vi "Update Values Buffer.vi"(8 "error in (no error)":errorcluster, 9 "buffer data":T1={"decimation"=0, "avg bandwidth"=0.0, "channels"=[], "byte order"=enum."little-endian", "buffer descriptor"={"buffer type"=enum."Engine", "plugin id"=0, "group id"=0, "transfer id"=0, "offset"=0, "length"=0}, "values channels"={"index"=0, "count"=0, "engine offset"=0}, "select start offset"=18446744073709551615, "select end offset"=0, "channel index"=-1} {"channels"."configuration"."string offset" format="%d bytes"; "avg bandwidth" format="%.0g bytes"}, 10 "buffer in":u8[](array[numeric]), 11 "values buffer in":u8[](array[numeric])) -> (0 "error out":errorcluster, 2 "buffer out":u8[](array[numeric]), 3 "values buffer out":u8[](array[numeric]))   [LabVIEW 2017, in "Data Viewer.lvlib"]
uses:
  Core/VIs/Data Viewer/Source/Data Viewer.lvlib
  Buffer Reader/Buffer Data.ctl
  VeriStand/Data Sharing Custom Device/Source/DSF Core.lvlibp/Classes/Configuration/Core/Transfer/Channel Configuration.ctl
  VeriStand/Data Sharing Custom Device/Source/DSF Core.lvlibp/Typedefs/Core Channel Configuration.ctl
  VeriStand/Data Sharing Custom Device/Source/DSF Core.lvlibp/Typedefs/DSF Data Type.ctl
  VeriStand/Data Sharing Custom Device/Source/DSF Core.lvlibp/Typedefs/DSF Settings Info.ctl
  VeriStand/Data Sharing Custom Device/Source/DSF Core.lvlibp/Typedefs/DSF Byte Order.ctl
  VeriStand/Data Sharing Custom Device/Source/DSF Core.lvlibp/Classes/Thread/Data Server/DSF Buffer Subset Descriptor.ctl
  VeriStand/Data Sharing Custom Device/Source/DSF Core.lvlibp/Typedefs/DSF Buffer Type.ctl
  Values Channels.ctl
  VeriStand/Data Sharing Custom Device/Source/DSF Core.lvlibp/Classes/Framework/Framework.lvclass
  VeriStand/Data Sharing Custom Device/Source/DSF Core.lvlibp
  VeriStand/Data Sharing Custom Device/Source/DSF Core.lvlibp/Classes/Configuration/Core/Channel/Channel Configuration.lvclass
  VeriStand/Data Sharing Custom Device/Source/DSF Core.lvlibp/Classes/Configuration/Core/Transfer/Transfer Configuration.lvclass
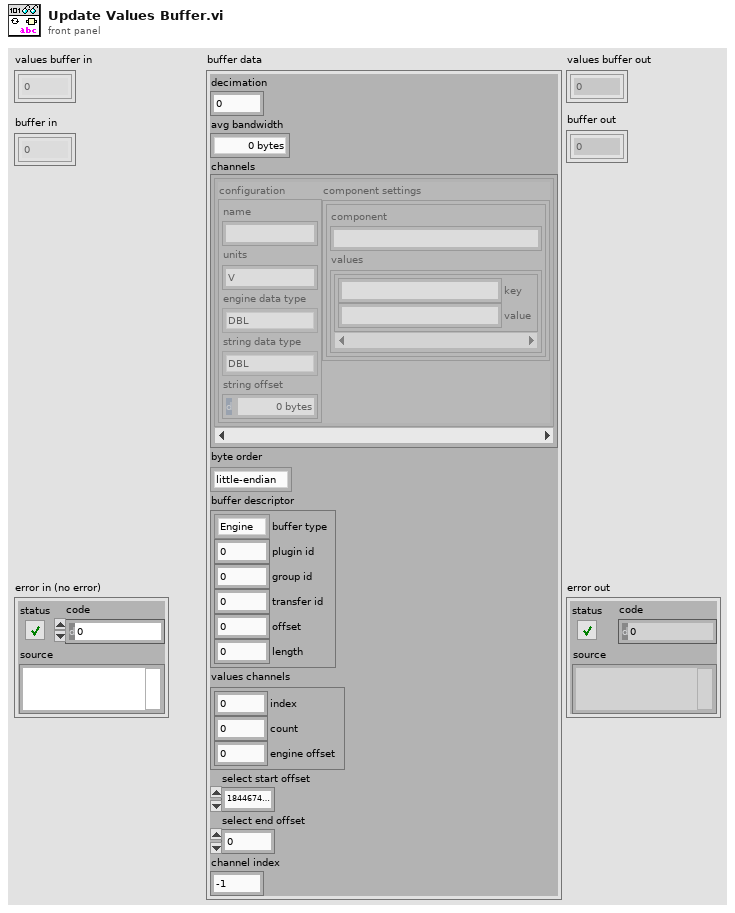
[diagram p1: front panel]
types:
  T1 = typedef "Data Viewer.lvlib/Buffer Data.ctl" = cluster{"decimation":u64, "avg bandwidth":dbl, "channels":T2[], "byte order":T6, "buffer descriptor":T7, "values channels":T9, "select start offset":u64, "select end offset":u64, "channel index":i32}
  T2 = typedef "DSF Core.lvlibp/Transfer Configuration.lvclass/Channel Configuration.ctl" = cluster{"configuration":T3, "component settings":T5[]}
  T3 = typedef "DSF Core.lvlibp/Channel Configuration.lvclass/Core Channel Configuration.ctl" = cluster{"name":string, "units":string, "engine data type":T4, "string data type":T4, "string offset":u64}
  T4 = typedef "DSF Core.lvlibp/DSF Data Type.ctl" = enum8{"Bool", "SGL", "DBL", "I8", "I16", "I32", "I64", "U8", "U16", "U32", "U64"}
  T5 = typedef "DSF Core.lvlibp/DSF Settings Info.ctl" = cluster{"component":string, "values":cluster{"key":string, "value":string}[]}
  T6 = typedef "DSF Core.lvlibp/DSF Byte Order.ctl" = enum8{"big-endian", "little-endian"}
  T7 = typedef "DSF Core.lvlibp/DSF Buffer Subset Descriptor.ctl" = cluster{"buffer type":T8, "plugin id":i32, "group id":i32, "transfer id":i32, "offset":u64, "length":i64}
  T8 = typedef "DSF Core.lvlibp/DSF Buffer Type.ctl" = enum16{"Engine", "String"}
  T9 = typedef "Data Viewer.lvlib/Values Channels.ctl" = cluster{"index":i32, "count":i32, "engine offset":u64}
  T10 = enum16{"big-endian, network order", "native, host order", "little-endian"}
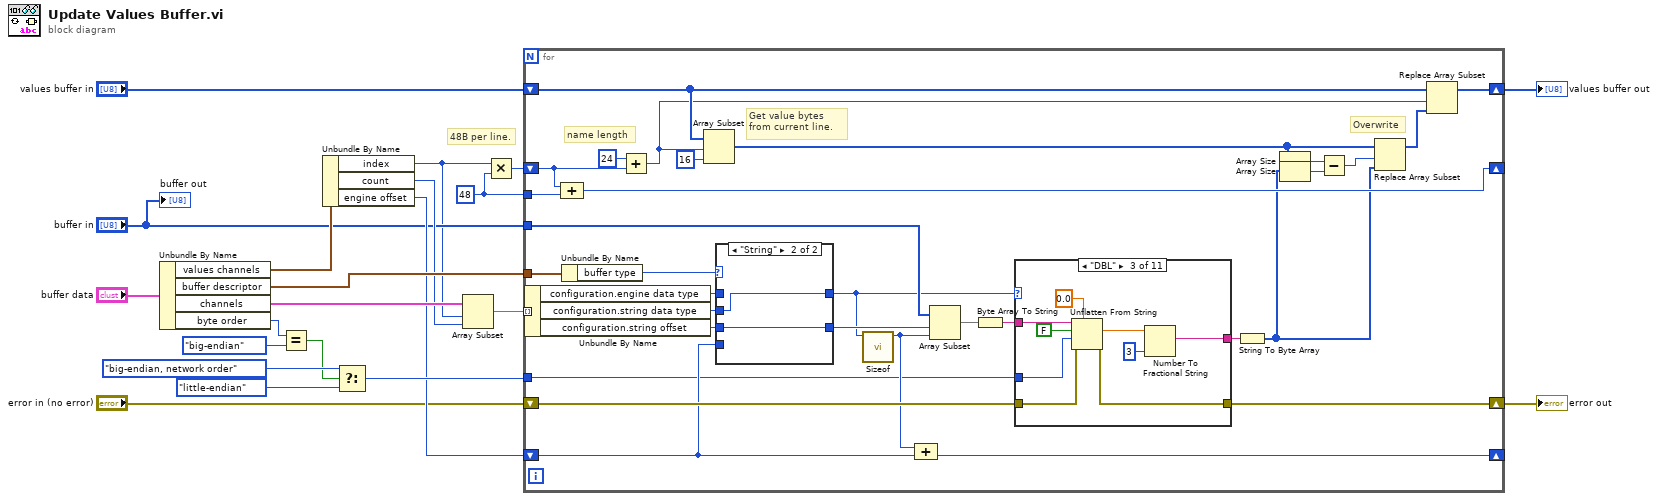
[diagram p0: block diagram]
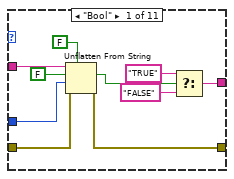
[diagram p3: hidden frame]
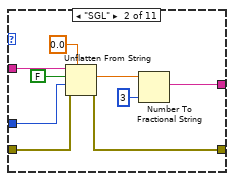
[diagram p4: hidden frame]
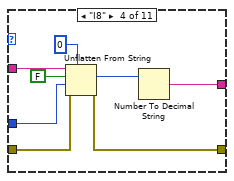
[diagram p5: hidden frame]
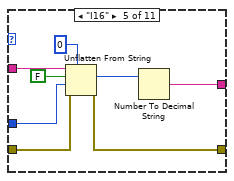
[diagram p6: hidden frame]
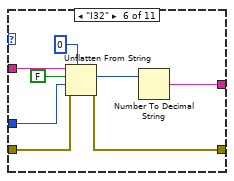
[diagram p7: hidden frame]
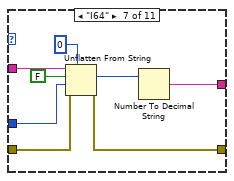
[diagram p8: hidden frame]
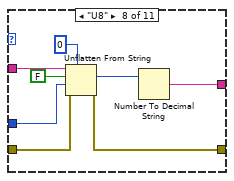
[diagram p9: hidden frame]
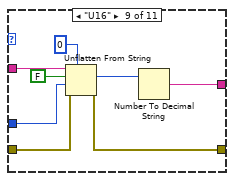
[diagram p10: hidden frame]
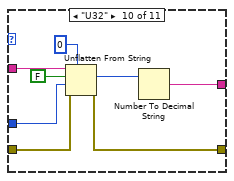
[diagram p11: hidden frame]
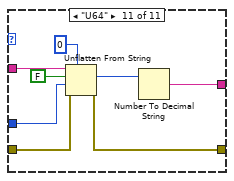
[diagram p12: hidden frame]
diagram:
  w1 = 48 ("x")
  # "48B per line."
  n1 = Unbundle By Name("buffer data") -> ("values channels"=w19:T9, "buffer descriptor"=w18:T7, "channels"=w17:T2[], "byte order"=w9:T6)
  n2 = Equal?(x=w9, y=DSF_Byte_Order."big-endian") -> (x = y?=w5:bool)
  n3 = Unbundle By Name(w19) -> ("index"=w2:i32, "count"=w10:i32, "engine offset"=w7:u64)
  n4 = Select(t=T10."big-endian, network order" ("byte order (0:big-endian, network order)"), s=w5, f=T10."little-endian") -> (s? t:f=w13:T10)
  n5 = Array Subset(array=w17, index=w2, length=w10) -> (w21:T2[])
  n6 = Multiply(x=w2, y=w1) -> (x*y=w3:i32)
  n7 = for {
    shift-right: [w29] -> w8
    shift-left: "error in (no error)" -> [w53]
    tunnel: w21 -> [w52] mode=indexing
    tunnel: w18 -> [w46]
    shift-right: [w47] -> _
    shift-left: w7 -> [w45]
    tunnel: w13 -> [w39]
    shift-right: [w43] -> w11
    shift-left: "values buffer in" -> [w44]
    tunnel: "buffer in" -> [w38]
    shift-right: [w30] -> _
    shift-left: w3 -> [w31]
    tunnel: w1 -> [w32]
    # "name length"
    # "Overwrite"
    # "Get value bytes from current line."
    n8 = Unbundle By Name(w52) -> ("configuration.engine data type"=w49:T4, "configuration.string data type"=w50:T4, "configuration.string offset"=w51:u64)
    n9 = Compound Arithmetic op=ADD(w31, w32) -> (w30:i32)
    n10 = Unbundle By Name(w46) -> ("buffer type"=w26:T8)
    n11 = Add(x=24, y=w31) -> (x+y=w40:i32)
    n12 = Array Subset(array=w44, index=w40, length=16) -> (w34:u8[])
    n13 = case shown="\"String\"" w26 {
      tunnel: w51 -> [_ w57]
      tunnel: [w54 w57] -> w28
      tunnel: w50 -> [_ w56]
      tunnel: w49 -> [w55 _]
      tunnel: w45 -> [w54 _]
      tunnel: [w55 w56] -> w27
      frame "Engine" {
      }
      frame "String" {
      }
    }
    n14 = call "Sizeof.vi"("data type"=w27) -> ("size in bytes"=w48:u64)  [unwired: 9 in, 1 out]
    n15 = Compound Arithmetic op=ADD(w48, w45) -> (w47:u64)
    n16 = Array Subset(array=w38, index=w28, length=w48) -> (w25:u8[])
    n17 = Byte Array To String(unsigned byte array=w25) -> (string=w24:string)
    n18 = case shown="\"DBL\"" w27 {
      tunnel: w53 -> [w67 w76 w85 w93 w101 w109 w117 w125 w133 w141 w149]
      tunnel: [w66 w75 w84 w92 w100 w108 w116 w124 w132 w140 w148] -> w29
      tunnel: w39 -> [w61 w72 w81 w89 w97 w105 w113 w121 w129 w137 w145]
      tunnel: [w60 w69 w78 w87 w95 w102 w111 w119 w127 w135 w143] -> w22
      tunnel: w24 -> [w58 w68 w77 w86 w94 w103 w110 w118 w126 w134 w142]
      frame "Bool" {
        n19 = Unflatten From String(type=FALSE, binary string=w58, data includes array or string size? (T)=FALSE, byte order (0:big-endian, network order)=w61, error in (no error)=w67) -> (value=w59:bool, error out=w66:errorcluster)  [unwired: 1 out]
        n20 = Select(t="TRUE", s=w59, f="FALSE") -> (s? t:f=w60:string)
      }
      frame "SGL" {
        n21 = Unflatten From String(type=sgl 0.0, binary string=w68, data includes array or string size? (T)=FALSE, byte order (0:big-endian, network order)=w72, error in (no error)=w76) -> (value=w70:sgl, error out=w75:errorcluster)  [unwired: 1 out]
        n22 = Number To Fractional String(number=w70, precision (6)=i16 3) -> (F-format string=w69:string)  [unwired: 2 in]
      }
      frame "DBL" {
        n23 = Unflatten From String(type=0.0, binary string=w77, data includes array or string size? (T)=FALSE, byte order (0:big-endian, network order)=w81, error in (no error)=w85) -> (value=w79:dbl, error out=w84:errorcluster)  [unwired: 1 out]
        n24 = Number To Fractional String(number=w79, precision (6)=i16 3) -> (F-format string=w78:string)  [unwired: 2 in]
      }
      frame "I8" {
        n25 = Unflatten From String(type=i8 0, binary string=w86, data includes array or string size? (T)=FALSE, byte order (0:big-endian, network order)=w89, error in (no error)=w93) -> (value=w88:i8, error out=w92:errorcluster)  [unwired: 1 out]
        n26 = Number To Decimal String(number=w88) -> (decimal integer string=w87:string)  [unwired: 1 in]
      }
      frame "I16" {
        n27 = Unflatten From String(type=i16 0, binary string=w94, data includes array or string size? (T)=FALSE, byte order (0:big-endian, network order)=w97, error in (no error)=w101) -> (value=w96:i16, error out=w100:errorcluster)  [unwired: 1 out]
        n28 = Number To Decimal String(number=w96) -> (decimal integer string=w95:string)  [unwired: 1 in]
      }
      frame "I32" {
        n29 = Unflatten From String(type=0, binary string=w103, data includes array or string size? (T)=FALSE, byte order (0:big-endian, network order)=w105, error in (no error)=w109) -> (value=w104:i32, error out=w108:errorcluster)  [unwired: 1 out]
        n30 = Number To Decimal String(number=w104) -> (decimal integer string=w102:string)  [unwired: 1 in]
      }
      frame "I64" {
        n31 = Unflatten From String(type=i64 0, binary string=w110, data includes array or string size? (T)=FALSE, byte order (0:big-endian, network order)=w113, error in (no error)=w117) -> (value=w112:i64, error out=w116:errorcluster)  [unwired: 1 out]
        n32 = Number To Decimal String(number=w112) -> (decimal integer string=w111:string)  [unwired: 1 in]
      }
      frame "U8" {
        n33 = Unflatten From String(type=u8 0, binary string=w118, data includes array or string size? (T)=FALSE, byte order (0:big-endian, network order)=w121, error in (no error)=w125) -> (value=w120:u8, error out=w124:errorcluster)  [unwired: 1 out]
        n34 = Number To Decimal String(number=w120) -> (decimal integer string=w119:string)  [unwired: 1 in]
      }
      frame "U16" {
        n35 = Unflatten From String(type=u16 0, binary string=w126, data includes array or string size? (T)=FALSE, byte order (0:big-endian, network order)=w129, error in (no error)=w133) -> (value=w128:u16, error out=w132:errorcluster)  [unwired: 1 out]
        n36 = Number To Decimal String(number=w128) -> (decimal integer string=w127:string)  [unwired: 1 in]
      }
      frame "U32" {
        n37 = Unflatten From String(type=u32 0, binary string=w134, data includes array or string size? (T)=FALSE, byte order (0:big-endian, network order)=w137, error in (no error)=w141) -> (value=w136:u32, error out=w140:errorcluster)  [unwired: 1 out]
        n38 = Number To Decimal String(number=w136) -> (decimal integer string=w135:string)  [unwired: 1 in]
      }
      frame "U64" {
        n39 = Unflatten From String(type=u64 0, binary string=w142, data includes array or string size? (T)=FALSE, byte order (0:big-endian, network order)=w145, error in (no error)=w149) -> (value=w144:u64, error out=w148:errorcluster)  [unwired: 1 out]
        n40 = Number To Decimal String(number=w144) -> (decimal integer string=w143:string)  [unwired: 1 in]
      }
    }
    n41 = String To Byte Array(string=w22) -> (unsigned byte array=w23:u8[])
    n42 = Array Size(array=w34) -> (size(s)=w37:i32)
    n43 = Array Size(array=w23) -> (size(s)=w36:i32)
    n44 = Subtract(x=w37, y=w36) -> (x-y=w35:i32)
    n45 = Replace Array Subset(array=w34, new element=w23, index=w35) -> (w33:u8[])
    n46 = Replace Array Subset(array=w44, new element=w33, index=w40) -> (w43:u8[])
  }
  "values buffer out" <- w11
  "error out" <- w8
  "buffer out" <- "buffer in"
